vi "AMC Multiple Targets Example 2 (RT).vi"() -> ()   [LabVIEW 2009]
uses:
  vi.lib/NI/AMC/AMC.lvlib
panel:
  in  "UDP Port":u16=9000
  in  "Exit":bool
  out "Process":bool
  out "Status":string
  in  "State Variables":cluster{"CurrentFile":path}
  # "Target 2"
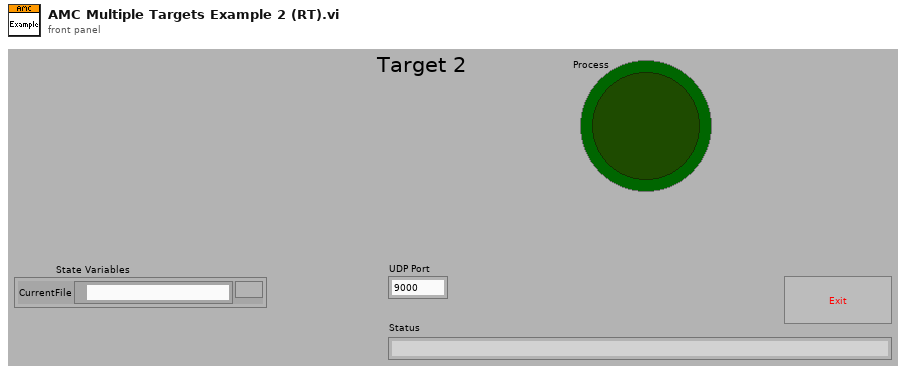
[diagram p1: front panel]
types:
  T1 = typedef "AMC.lvlib/Message Queue.ctl" = refnum<queue>
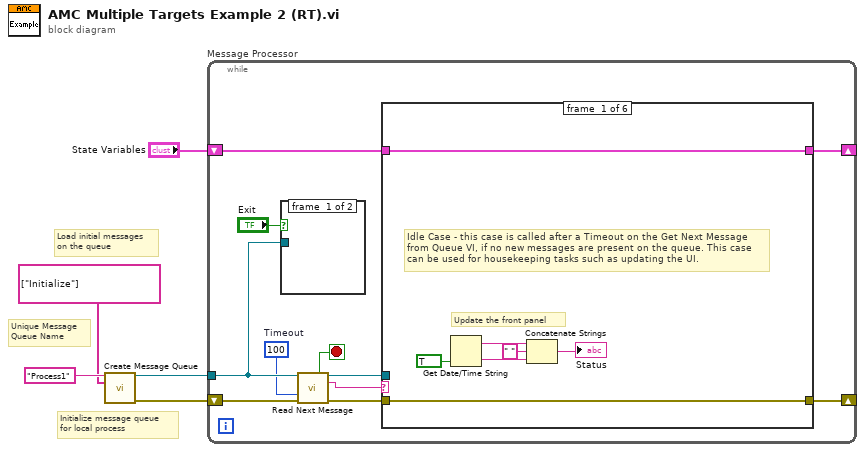
[diagram p0: block diagram]
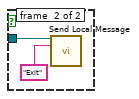
[diagram p2: hidden frame]
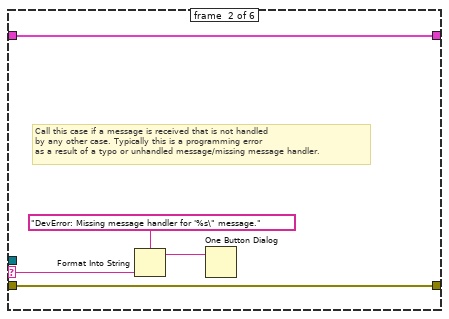
[diagram p3: hidden frame]
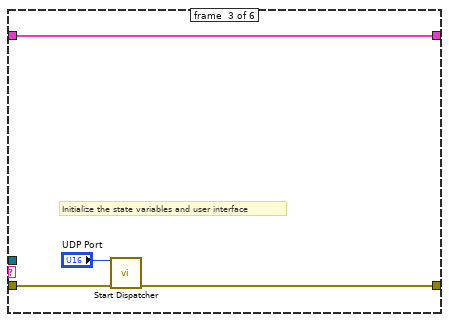
[diagram p4: hidden frame]
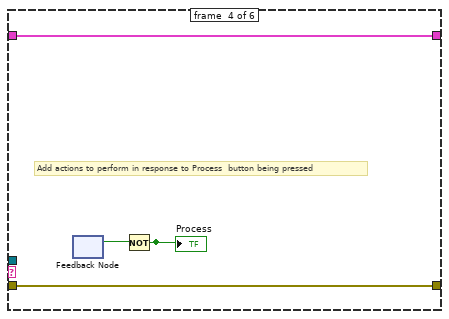
[diagram p5: hidden frame]
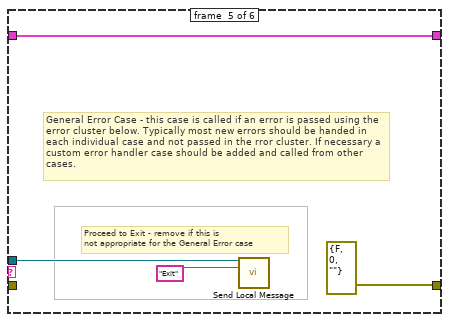
[diagram p6: hidden frame]
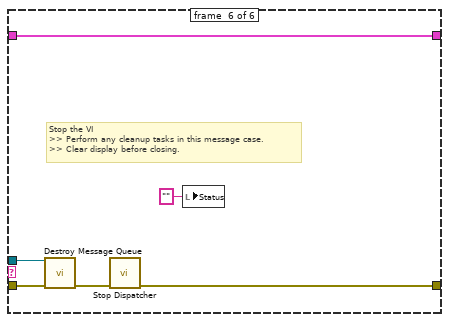
[diagram p7: hidden frame]
diagram:
  # "Initialize message queue\nfor local process"
  # "Unique Message\nQueue Name"
  # "Load initial messages\non the queue"
  n1 = call "Create Message Queue.vi"("message queue name"="Process1" ("Message queue name (unnamed)"), "initial message names"=string[] ["Initialize"]) -> ("message queue out"=w4:T1, "error out"=w2:errorcluster)  [unwired: 12 in]
  n2 = while "Message Processor" {
    shift-left: w2 -> [w11]
    shift-right: [w12] -> _
    tunnel: w4 -> [w7]
    shift-left: "State Variables" -> [w16]
    shift-right: [w15] -> _
    stop <- w9 stop-if-true
    w6 = 100  # Timeout
    n3 = case shown="True" "Exit" {
      tunnel: w7 -> [_ w17]
      frame #0 {
      }
      frame #1 {
        n4 = call "Send Local Message.vi"("message queue in"=w17, "message name"="Exit") -> ()  [unwired: 11 in, 3 out]
      }
    }
    n5 = call "Read Next Message.vi"("message queue in"=w7, "timeout (1 ms)"=w6, "error in"=w11) -> ("exit process?"=w9:bool, "message queue out"=w14:T1, "message name"=w10:string, "error out"=w13:errorcluster)  [unwired: 5 in, 4 out]
    n6 = case shown="\"Initialize\"" w10 {
      selector: w10 -> [_ w28 _ _ _ _]
      tunnel: [w25 w30 w34 w37 w42 w48] -> w15
      tunnel: w16 -> [w25 w30 w34 w37 w42 w48]
      tunnel: w14 -> [_ _ _ _ w40 w46]
      tunnel: w13 -> [w24 w29 w33 w38 _ w45]
      tunnel: [w24 w29 w32 w38 errorcluster {"status"=FALSE, "code"=0, "source"=""} ("error out") w43] -> w12
      frame #0 {
        # "Update the front panel"
        # "Idle Case - this case is called after a Timeout on the Get Next Message from Queue VI, if no new messages are present on the queue. This case can be used for housekeeping tasks such as updating the UI."
        n7 = Get Date/Time String(want seconds? (F)=TRUE) -> (date string=w23:string, time string=w22:string)  [unwired: 2 out]
        n8 = Concatenate Strings(w23, " " ("string"), w22) -> (→"Status":string)
      }
      frame #1 {
        # "Call this case if a message is received that is not handled \nby any other case. Typically this is a programming error\nas a result of a typo or unhandled message/missing message handler."
        n9 = Format Into String(format string="DevError: Missing message handler for '%s\" message." ("message"), w28) -> (resulting string=w26:string)  [unwired: 2 in, 1 out]
        n10 = One Button Dialog(message=w26) -> ()  [unwired: 2 out]
      }
      frame #2 {
        # "Initialize the state variables and user interface"
        n11 = call "Start Dispatcher.vi"("UDP port (0)"="UDP Port", "error in"=w33) -> ("error out"=w32:errorcluster)  [unwired: 11 in, 2 out]
      }
      frame #3 {
        # "Add actions to perform in response to Process  button being pressed"
        n12 = feedback #1() -> (w36:bool)  [unwired: 1 out]
        n13 = Not(x=w36) -> (.not. x?=w35:bool)
        "Process" <- w35
      }
      frame #4 {
        # "Proceed to Exit - remove if this is\nnot appropriate for the General Error case"
        # "General Error Case - this case is called if an error is passed using the error cluster below. Typically most new errors should be handed in each individual case and not passed in the rror cluster. If necessary a custom error handler case should be added and called from other cases."
        n14 = call "Send Local Message.vi"("message queue in"=w40, "message name"="Exit") -> ()  [unwired: 11 in, 3 out]
      }
      frame #5 {
        # "Stop the VI\n>> Perform any cleanup tasks in this message case.\n>> Clear display before closing."
        n15 = call "Destroy Message Queue.vi"("message queue in"=w46, "error in"=w45) -> ("error out"=w44:errorcluster)  [unwired: 11 in, 2 out]
        n16 = call "Stop Dispatcher.vi"("error in"=w44) -> ("error out"=w43:errorcluster)  [unwired: 14 in]
        n17 = local write "Status"("" ("Status")) -> ()
      }
    }
  }
